vi "Main.vi"() -> ()   [LabVIEW 2017]
uses:
  Variable globale.vi
  Settings/Traverse-Settings-Global.vi
  ICNC/ICNC2.lvlib
panel:
  in  "Go Relative":bool
  out "Speed Z":dbl
  out "Speed X":dbl
  out "Speed Y":dbl
  in  "Load Settings":bool
  in  "x-":bool
  in  "x+":bool
  in  "z+":bool
  in  "z-":bool
  in  "y+":bool
  in  "y-":bool
  in  "z+y+":bool
  in  "z-y+":bool
  in  "z-y-":bool
  in  "z+y-":bool
  in  "Speed in mm/s":dbl(slide) scale=0.0..150.0
  in  "Go Absolute":bool
  in  "Z":dbl
  in  "Y":dbl
  in  "X":dbl
  in  "System settings":bool
  out "Unlocked":bool
  out "Connected":bool
  in  "PARAM DLG":bool
  in  "stop motors":bool
  in  "Pos0":bool
  in  "stop":bool
  # "POSITION"
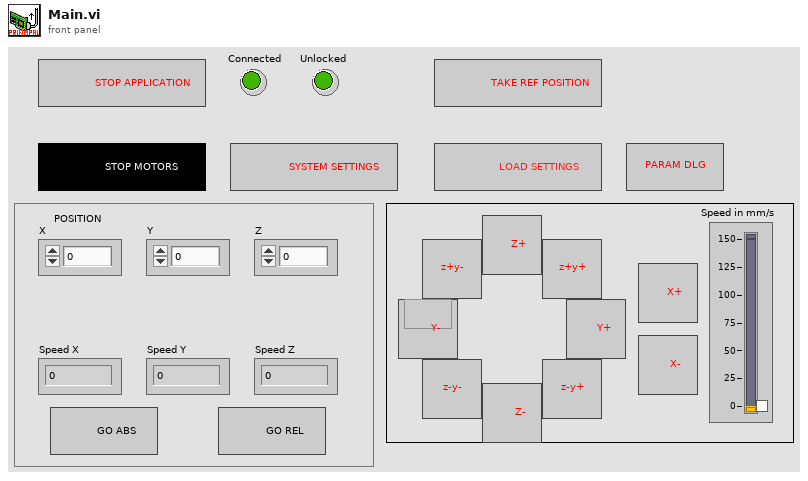
[diagram p1: front panel]
types:
  T1 = typedef "Settings-Control.ctl" = cluster{"Acceleration":dbl[], "Deceleration":dbl[], "Max Velocity":dbl[], "Speed":dbl, "Pulse/Degree":dbl, "Degre Factor":dbl[], "mm/rotation":dbl[], "Traverse Name":string}
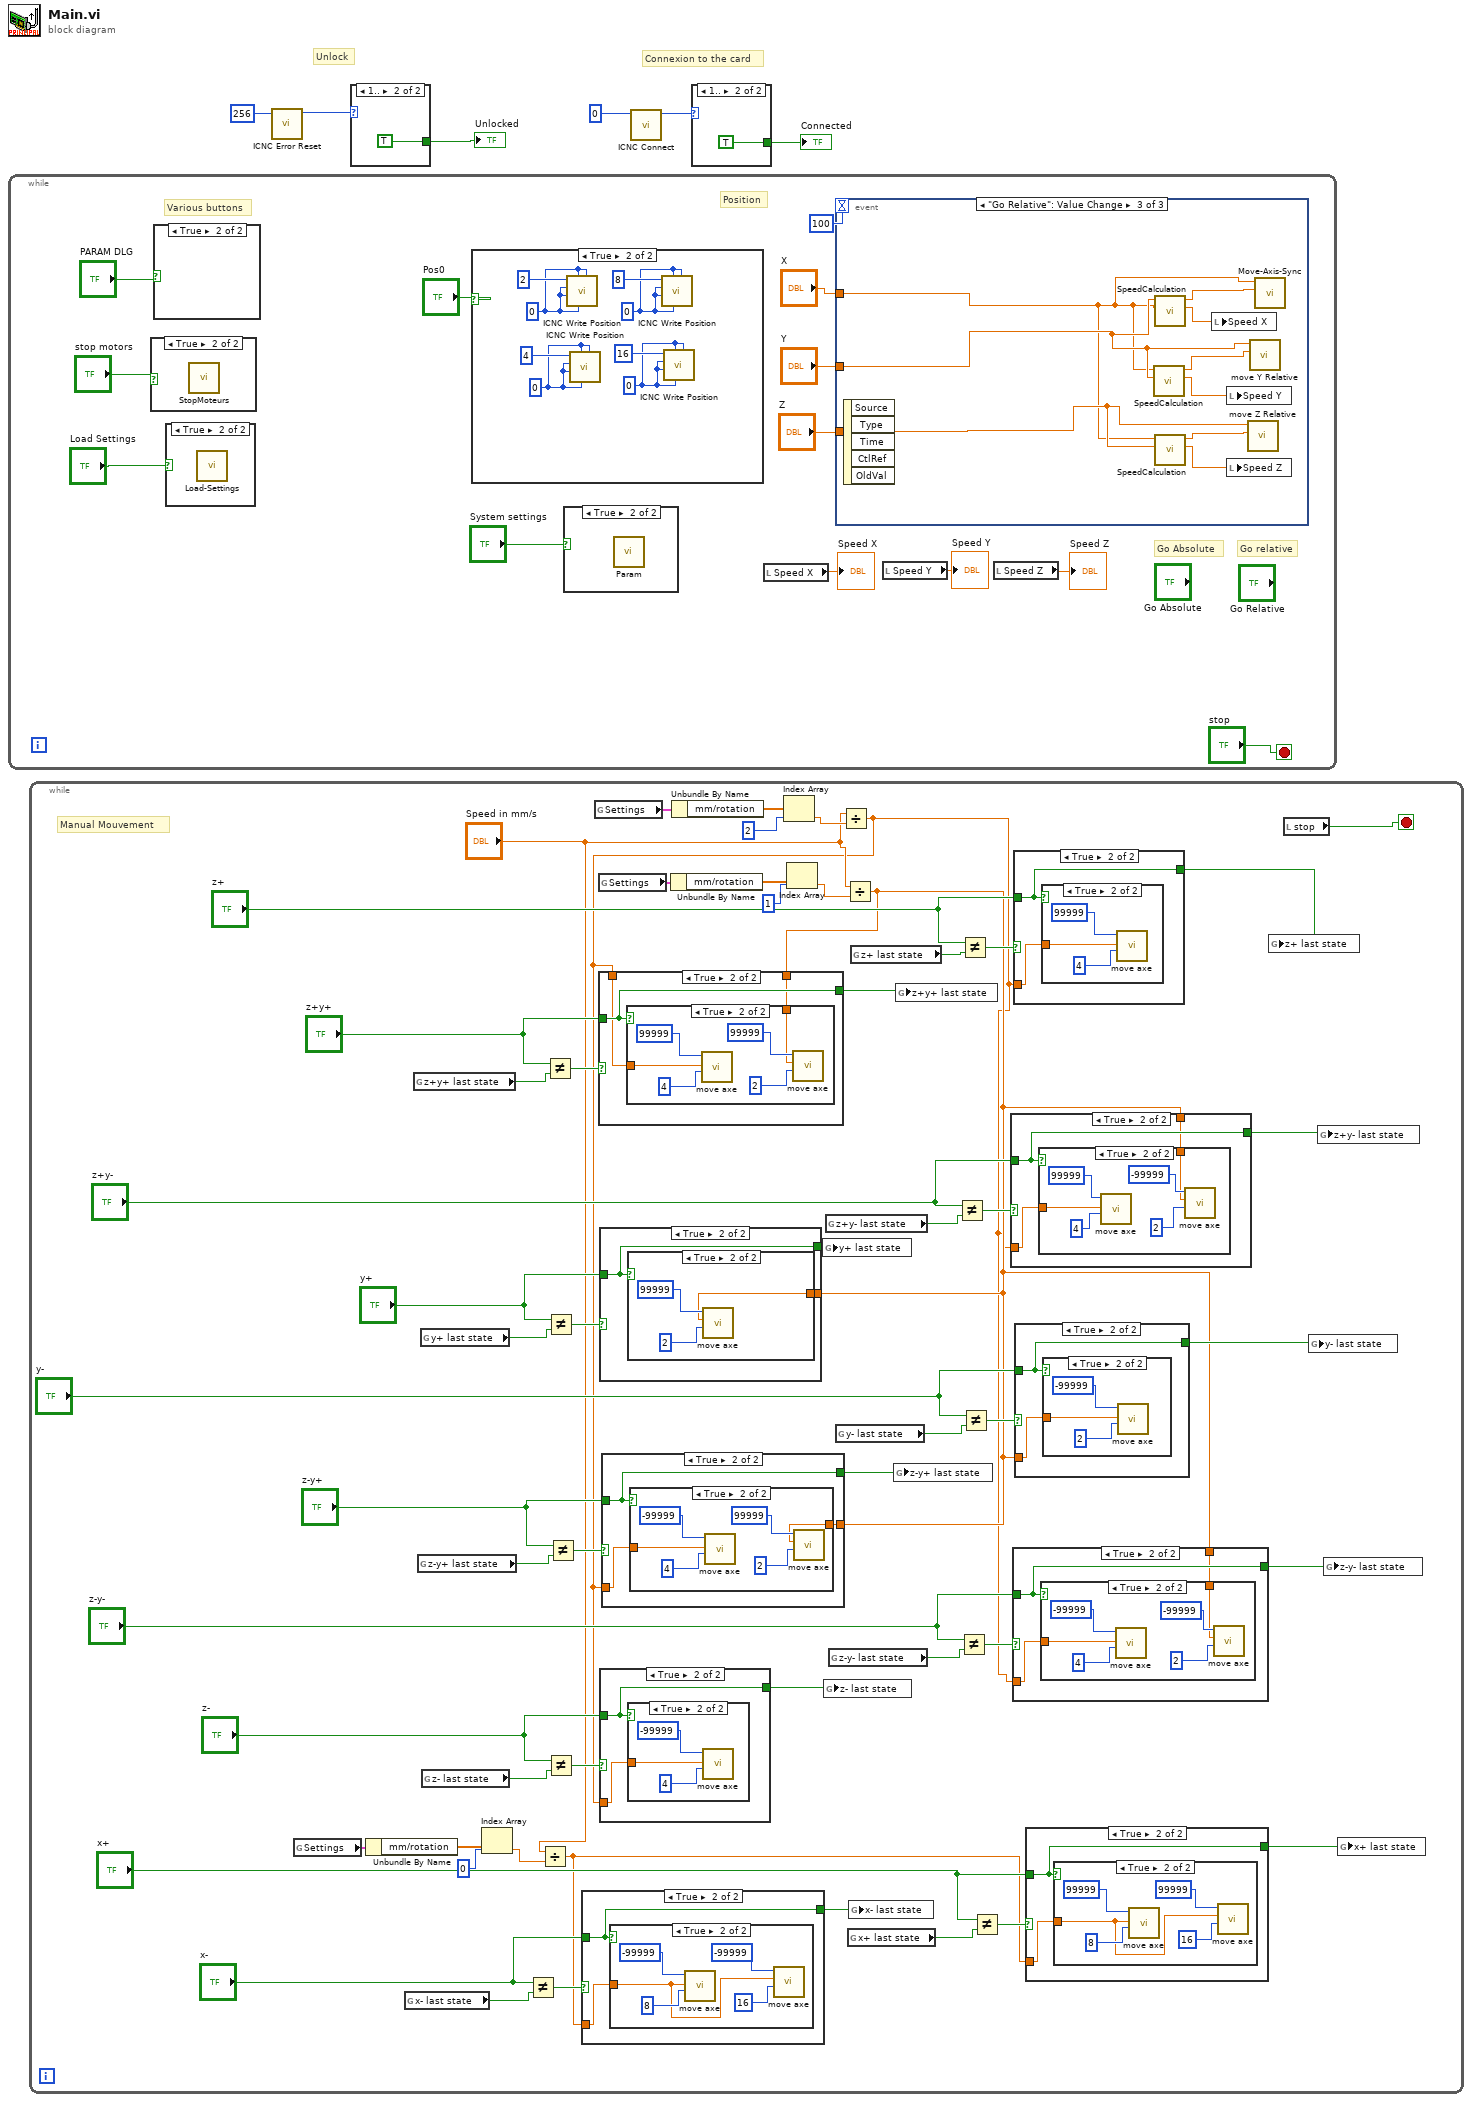
[diagram p0: block diagram]
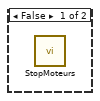
[diagram p3: hidden frame]
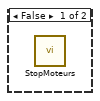
[diagram p5: hidden frame]
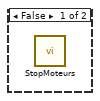
[diagram p7: hidden frame]
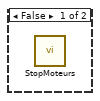
[diagram p9: hidden frame]
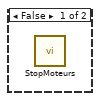
[diagram p11: hidden frame]
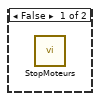
[diagram p13: hidden frame]
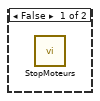
[diagram p15: hidden frame]
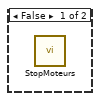
[diagram p17: hidden frame]
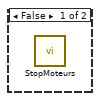
[diagram p19: hidden frame]
diagram:
  # "Connexion to the card"
  # "Unlock"
  n1 = while {
    stop <- "stop" stop-if-true
    # "Go relative"
    # "Go Absolute"
    # "Various buttons"
    # "Position"
    n2 = case shown="True" "stop motors" {
      frame False {
      }
      frame True {
        n3 = call "StopMoteurs.vi"() -> ()  [unwired: 12 in]
      }
    }
    n4 = case shown="True" "PARAM DLG" {
      frame False {
      }
      frame True {
      }
    }
    n5 = case shown="True" "Load Settings" {
      frame False {
      }
      frame True {
        n6 = call "Load-Settings.vi"() -> ()  [unwired: 12 in]
      }
    }
    n7 = case shown="True" "Pos0" {
      frame False {
      }
      frame True {
        w21 = 0
        w20 = 0
        w24 = 0
        w26 = 0
        n8 = call "ICNC Write Position.vi"("PositionB"=w26, "PositionA"=w26, "PositionZ"=w26, "PositionY"=w26, "PositionX"=w26, "Axis"=2) -> ()  [unwired: 4 in, 2 out]
        n9 = call "ICNC Write Position.vi"("PositionB"=w24, "PositionA"=w24, "PositionZ"=w24, "PositionY"=w24, "PositionX"=w24, "Axis"=4) -> ()  [unwired: 4 in, 2 out]
        n10 = call "ICNC Write Position.vi"("PositionB"=w20, "PositionA"=w20, "PositionZ"=w20, "PositionY"=w20, "PositionX"=w20, "Axis"=8) -> ()  [unwired: 4 in, 2 out]
        n11 = call "ICNC Write Position.vi"("PositionB"=w21, "PositionA"=w21, "PositionZ"=w21, "PositionY"=w21, "PositionX"=w21, "Axis"=16) -> ()  [unwired: 4 in, 2 out]
      }
    }
    n12 = case shown="True" "System settings" {
      frame False {
      }
      frame True {
        n13 = call "Param.vi"() -> ()  [unwired: 12 in]
      }
    }
    n14 = local read "Speed X"() -> (→"Speed X":dbl)
    n15 = event shown="[2] \"Go Relative\": Value Change" {
      selector: _ -> [_ _ _]
      dyn-events: _ -> [_ _ _]
      timeout: 100 -> [_ _ _]
      tunnel: "X" -> [_ w30 w38]
      tunnel: "Y" -> [_ w28 w42]
      tunnel: "Z" -> [_ w29 w43]
      event Timeout {
        n16 = event-data() -> ()  [unwired: 1 in, 2 out]
      }
      event "Go Absolute": Value Change {
        n17 = event-data() -> ()  [unwired: 1 in, 5 out]
        n18 = call "SpeedCalculation.vi"("Axis1"=w28, "Axis2"=w30) -> ("Speed mm/s"=w32:dbl, "Speed for card"=w36:dbl)  [unwired: 8 in]
        n19 = call "SpeedCalculation.vi"("Axis1"=w30, "Axis2"=w28) -> ("Speed mm/s"=w33:dbl, "Speed for card"=w35:dbl)  [unwired: 8 in]
        n20 = call "SpeedCalculation.vi"("Axis1"=w29, "Axis2"=w30) -> ("Speed mm/s"=w31:dbl, "Speed for card"=w34:dbl)  [unwired: 8 in]
        n21 = call "move X.vi"("Speed X"=w35, "x mm"=w30) -> ()  [unwired: 10 in]
        n22 = call "move Y.vi"("Y Speed"=w36, "y mm"=w28) -> ()  [unwired: 10 in]
        n23 = call "move Z.vi"("Z Speed"=w34, "z mm"=w29) -> ()  [unwired: 10 in]
        n24 = local write "Speed X"(w33) -> ()
        n25 = local write "Speed Z"(w31) -> ()
        n26 = local write "Speed Y"(w32) -> ()
      }
      event "Go Relative": Value Change {
        n27 = event-data() -> ()  [unwired: 1 in, 5 out]
        n28 = call "SpeedCalculation.vi"("Axis1"=w42, "Axis2"=w38) -> ("Speed mm/s"=w40:dbl, "Speed for card"=w44:dbl)  [unwired: 8 in]
        n29 = call "SpeedCalculation.vi"("Axis1"=w38, "Axis2"=w42) -> ("Speed mm/s"=w41:dbl, "Speed for card"=w37:dbl)  [unwired: 8 in]
        n30 = call "SpeedCalculation.vi"("Axis1"=w43, "Axis2"=w38) -> ("Speed mm/s"=w39:dbl, "Speed for card"=w45:dbl)  [unwired: 8 in]
        n31 = local write "Speed X"(w41) -> ()
        n32 = local write "Speed Y"(w40) -> ()
        n33 = local write "Speed Z"(w39) -> ()
        n34 = call "move Z Relative.vi"("Z Speed"=w45, "z mm"=w43) -> ()  [unwired: 10 in]
        n35 = call "move Y Relative.vi"("Y Speed"=w44, "y mm"=w42) -> ()  [unwired: 10 in]
        n36 = call "Move-Axis-Sync.vi"("Speed X"=w37, "x mm"=w38) -> ()  [unwired: 10 in]
      }
    }
    n37 = local read "Speed Y"() -> (→"Speed Y":dbl)
    n38 = local read "Speed Z"() -> (→"Speed Z":dbl)
  }
  n39 = while {
    stop <- w70 stop-if-true
    # "Manual Mouvement"
    n40 = global read "Traverse-Settings-Global.vi" "Settings"() -> (w61:T1)
    n41 = Unbundle By Name(w61) -> ("mm/rotation"=w60:dbl[])
    n42 = global read "Variable globale.vi" "x- last state"() -> (w64:bool)
    n43 = global read "Variable globale.vi" "z+y+ last state"() -> (w97:bool)
    n44 = global read "Variable globale.vi" "z-y+ last state"() -> (w81:bool)
    n45 = global read "Variable globale.vi" "y+ last state"() -> (w89:bool)
    n46 = global read "Variable globale.vi" "z- last state"() -> (w93:bool)
    n47 = Index Array(array=w60, index=0) -> (element=w58:dbl)
    n48 = Not Equal?(x="x-", y=w64) -> (x != y?=w65:bool)
    n49 = Divide(x="Speed in mm/s", y=w58) -> (x/y=w57:dbl)
    n50 = Not Equal?(x="z+y+", y=w97) -> (x != y?=w98:bool)
    n51 = Not Equal?(x="y+", y=w89) -> (x != y?=w90:bool)
    n52 = Not Equal?(x="z-", y=w93) -> (x != y?=w94:bool)
    n53 = Not Equal?(x="z-y+", y=w81) -> (x != y?=w82:bool)
    n54 = case shown="True" w65 {
      tunnel: w57 -> [_ w105]
      tunnel: "x-" -> [w103 w104]
      tunnel: [w103 w104] -> w63
      frame False {
      }
      frame True {
        n55 = case shown="True" w104 {
          tunnel: w105 -> [_ w106]
          frame False {
            n56 = call "StopMoteurs.vi"() -> ()  [unwired: 12 in]
          }
          frame True {
            n57 = call "move axe.vi"("Axe"=8, "Speed"=w106, "Angle"=-99999) -> ()  [unwired: 9 in]
            n58 = call "move axe.vi"("Axe"=16, "Speed"=w106, "Angle"=-99999) -> ()  [unwired: 9 in]
          }
        }
      }
    }
    n59 = global read "Traverse-Settings-Global.vi" "Settings"() -> (w51:T1)
    n60 = global read "Traverse-Settings-Global.vi" "Settings"() -> (w56:T1)
    n61 = Unbundle By Name(w56) -> ("mm/rotation"=w55:dbl[])
    n62 = Unbundle By Name(w51) -> ("mm/rotation"=w50:dbl[])
    n63 = Index Array(array=w50, index=2) -> (element=w48:dbl)
    n64 = Index Array(array=w55, index=1) -> (element=w53:dbl)
    n65 = global read "Variable globale.vi" "z+y- last state"() -> (w85:bool)
    n66 = global read "Variable globale.vi" "z-y- last state"() -> (w73:bool)
    n67 = global read "Variable globale.vi" "y- last state"() -> (w77:bool)
    n68 = Divide(x="Speed in mm/s", y=w48) -> (x/y=w46:dbl)
    n69 = case shown="True" w94 {
      tunnel: w46 -> [_ w163]
      tunnel: "z-" -> [w161 w162]
      tunnel: [w161 w162] -> w92
      frame False {
      }
      frame True {
        n70 = case shown="True" w162 {
          tunnel: w163 -> [_ w165]
          frame False {
            n71 = call "StopMoteurs.vi"() -> ()  [unwired: 12 in]
          }
          frame True {
            n72 = call "move axe.vi"("Axe"=4, "Speed"=w165, "Angle"=-99999) -> ()  [unwired: 9 in]
          }
        }
      }
    }
    n73 = global write "Variable globale.vi" "z- last state"(w92) -> ()
    n74 = Divide(x="Speed in mm/s", y=w53) -> (x/y=w52:dbl)
    n75 = case shown="True" w98 {
      tunnel: "z+y+" -> [w167 w170]
      tunnel: [w167 w170] -> w96
      tunnel: w52 -> [_ w169]
      tunnel: w46 -> [_ w168]
      frame False {
      }
      frame True {
        n76 = case shown="True" w170 {
          tunnel: w168 -> [_ w173]
          tunnel: w169 -> [_ w171]
          frame False {
            n77 = call "StopMoteurs.vi"() -> ()  [unwired: 12 in]
          }
          frame True {
            n78 = call "move axe.vi"("Axe"=4, "Speed"=w173, "Angle"=99999) -> ()  [unwired: 9 in]
            n79 = call "move axe.vi"("Axe"=2, "Speed"=w171, "Angle"=99999) -> ()  [unwired: 9 in]
          }
        }
      }
    }
    n80 = case shown="True" w90 {
      tunnel: "y+" -> [w155 w157]
      tunnel: [w155 w157] -> w88
      tunnel: w52 -> [_ w156]
      frame False {
      }
      frame True {
        n81 = case shown="True" w157 {
          tunnel: w156 -> [_ w158]
          frame False {
            n82 = call "StopMoteurs.vi"() -> ()  [unwired: 12 in]
          }
          frame True {
            n83 = call "move axe.vi"("Axe"=2, "Speed"=w158, "Angle"=99999) -> ()  [unwired: 9 in]
          }
        }
      }
    }
    n84 = case shown="True" w82 {
      tunnel: w46 -> [_ w138]
      tunnel: "z-y+" -> [w135 w137]
      tunnel: [w135 w137] -> w80
      tunnel: w52 -> [_ w136]
      frame False {
      }
      frame True {
        n85 = case shown="True" w137 {
          tunnel: w138 -> [_ w139]
          tunnel: w136 -> [_ w140]
          frame False {
            n86 = call "StopMoteurs.vi"() -> ()  [unwired: 12 in]
          }
          frame True {
            n87 = call "move axe.vi"("Axe"=4, "Speed"=w139, "Angle"=-99999) -> ()  [unwired: 9 in]
            n88 = call "move axe.vi"("Axe"=2, "Speed"=w140, "Angle"=99999) -> ()  [unwired: 9 in]
          }
        }
      }
    }
    n89 = global write "Variable globale.vi" "y+ last state"(w88) -> ()
    n90 = global read "Variable globale.vi" "x+ last state"() -> (w68:bool)
    n91 = global write "Variable globale.vi" "x- last state"(w63) -> ()
    n92 = global read "Variable globale.vi" "z+ last state"() -> (w101:bool)
    n93 = global write "Variable globale.vi" "z-y+ last state"(w80) -> ()
    n94 = global write "Variable globale.vi" "z+y+ last state"(w96) -> ()
    n95 = Not Equal?(x="z+y-", y=w85) -> (x != y?=w86:bool)
    n96 = Not Equal?(x="z-y-", y=w73) -> (x != y?=w74:bool)
    n97 = Not Equal?(x="z+", y=w101) -> (x != y?=w102:bool)
    n98 = Not Equal?(x="y-", y=w77) -> (x != y?=w78:bool)
    n99 = Not Equal?(x="x+", y=w68) -> (x != y?=w69:bool)
    n100 = case shown="True" w86 {
      tunnel: w46 -> [_ w148]
      tunnel: "z+y-" -> [w145 w147]
      tunnel: [w145 w147] -> w84
      tunnel: w52 -> [_ w146]
      frame False {
      }
      frame True {
        n101 = case shown="True" w147 {
          tunnel: w148 -> [_ w150]
          tunnel: w146 -> [_ w149]
          frame False {
            n102 = call "StopMoteurs.vi"() -> ()  [unwired: 12 in]
          }
          frame True {
            n103 = call "move axe.vi"("Axe"=4, "Speed"=w150, "Angle"=99999) -> ()  [unwired: 9 in]
            n104 = call "move axe.vi"("Axe"=2, "Speed"=w149, "Angle"=-99999) -> ()  [unwired: 9 in]
          }
        }
      }
    }
    n105 = case shown="True" w74 {
      tunnel: w46 -> [_ w122]
      tunnel: "z-y-" -> [w119 w121]
      tunnel: [w119 w121] -> w72
      tunnel: w52 -> [_ w120]
      frame False {
      }
      frame True {
        n106 = case shown="True" w121 {
          tunnel: w122 -> [_ w124]
          tunnel: w120 -> [_ w123]
          frame False {
            n107 = call "StopMoteurs.vi"() -> ()  [unwired: 12 in]
          }
          frame True {
            n108 = call "move axe.vi"("Axe"=4, "Speed"=w124, "Angle"=-99999) -> ()  [unwired: 9 in]
            n109 = call "move axe.vi"("Axe"=2, "Speed"=w123, "Angle"=-99999) -> ()  [unwired: 9 in]
          }
        }
      }
    }
    n110 = case shown="True" w102 {
      tunnel: w46 -> [_ w179]
      tunnel: "z+" -> [w177 w178]
      tunnel: [w177 w178] -> w100
      frame False {
      }
      frame True {
        n111 = case shown="True" w178 {
          tunnel: w179 -> [_ w181]
          frame False {
            n112 = call "StopMoteurs.vi"() -> ()  [unwired: 12 in]
          }
          frame True {
            n113 = call "move axe.vi"("Axe"=4, "Speed"=w181, "Angle"=99999) -> ()  [unwired: 9 in]
          }
        }
      }
    }
    n114 = case shown="True" w78 {
      tunnel: w52 -> [_ w131]
      tunnel: "y-" -> [w129 w130]
      tunnel: [w129 w130] -> w76
      frame False {
      }
      frame True {
        n115 = case shown="True" w130 {
          tunnel: w131 -> [_ w133]
          frame False {
            n116 = call "StopMoteurs.vi"() -> ()  [unwired: 12 in]
          }
          frame True {
            n117 = call "move axe.vi"("Axe"=2, "Speed"=w133, "Angle"=-99999) -> ()  [unwired: 9 in]
          }
        }
      }
    }
    n118 = case shown="True" w69 {
      tunnel: w57 -> [_ w113]
      tunnel: "x+" -> [w111 w112]
      tunnel: [w111 w112] -> w67
      frame False {
      }
      frame True {
        n119 = case shown="True" w112 {
          tunnel: w113 -> [_ w114]
          frame False {
            n120 = call "StopMoteurs.vi"() -> ()  [unwired: 12 in]
          }
          frame True {
            n121 = call "move axe.vi"("Axe"=8, "Speed"=w114, "Angle"=99999) -> ()  [unwired: 9 in]
            n122 = call "move axe.vi"("Axe"=16, "Speed"=w114, "Angle"=99999) -> ()  [unwired: 9 in]
          }
        }
      }
    }
    n123 = global write "Variable globale.vi" "z+ last state"(w100) -> ()
    n124 = local read "stop"() -> (w70:bool)
    n125 = global write "Variable globale.vi" "y- last state"(w76) -> ()
    n126 = global write "Variable globale.vi" "z+y- last state"(w84) -> ()
    n127 = global write "Variable globale.vi" "z-y- last state"(w72) -> ()
    n128 = global write "Variable globale.vi" "x+ last state"(w67) -> ()
  }
  n129 = call "ICNC Error Reset.vi"("ErrorBits"=256) -> ("function return"=w2:u32)  [unwired: 9 in, 1 out]
  n130 = case shown="1.." w2 {
    tunnel: [FALSE TRUE] -> w5
    frame ..0 {
    }
    frame 1.. {
    }
  }
  "Unlocked" <- w5
  n131 = call "ICNC Connect.vi"("ICNC_Number"=0) -> ("function return"=w3:u32)  [unwired: 9 in, 1 out]
  n132 = case shown="1.." w3 {
    tunnel: [FALSE TRUE] -> w6
    frame ..0 {
    }
    frame 1.. {
    }
  }
  "Connected" <- w6
